vi "Configure Harmonics Fetch Step.vi"(6 "SA Pin":string="SA PIN", 8 "error in (no error)":errorcluster, 9 "Result Name":string, 10 "Harmonic Order":i8, 11 "Harmonics in":refnum<class "Harmonics.lvclass">) -> (0 "error out":errorcluster, 2 "Exported Data Location":string, 3 "Harmonics out":refnum<class "Harmonics.lvclass">)   [LabVIEW 2018, in "Harmonics.lvlib" / "Harmonics.lvclass"]
uses:
  Harmonics.lvclass
  C:/Sequence Automation/Plugins/Measurement Interface.lvlibp/Measurement Interface.lvclass
  Plugins/Measurement Interface.lvlibp/Private Methods/Engine Reference/Read Engine Reference.vi
  Plugins/Measurement Interface.lvlibp/Private Methods/Measurement Name/Read Measurement Name.vi
  Plugins/Measurement Interface.lvlibp/Public Methods/Sequence Reference/Read Sequence Reference.vi
  Plugins/TestStand API Tools (TSAT).lvlibp/Step Actions/TSAT Step Actions.lvlib
  Plugins/TestStand API Tools (TSAT).lvlibp/Sequence Actions/TSAT Sequence Actions.lvlib
  Plugins/Measurement Interface.lvlibp/Measurement Interface.lvclass
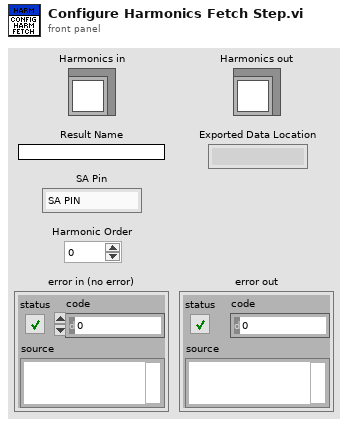
[diagram p1: front panel]
types:
  T1 = typedef "TestStand API Tools (TSAT).lvlibp/TSAT Evaluation Actions.lvlib/TSAT Evaluation.ctl" = cluster{"Test Name":string, "Pin":string, "Units":string, "SI Scaling":T2, "Test Number":i32, "Published Data Id":string, "Low Limit":dbl, "High Limit":dbl, "Export Data Location":string, "Software Bin":i64, "Evaluation Type":T3, "Test Data Source":string}
  T2 = typedef "TestStand API Tools (TSAT).lvlibp/TSAT Evaluation Actions.lvlib/TSAT Eval SI Unit Scaling.ctl" = i16
  T3 = typedef "TestStand API Tools (TSAT).lvlibp/TSAT Evaluation Actions.lvlib/TSAT Evaluation Type.ctl" = enum16{"Numeric Limit", "Pass/Fail", "None"}
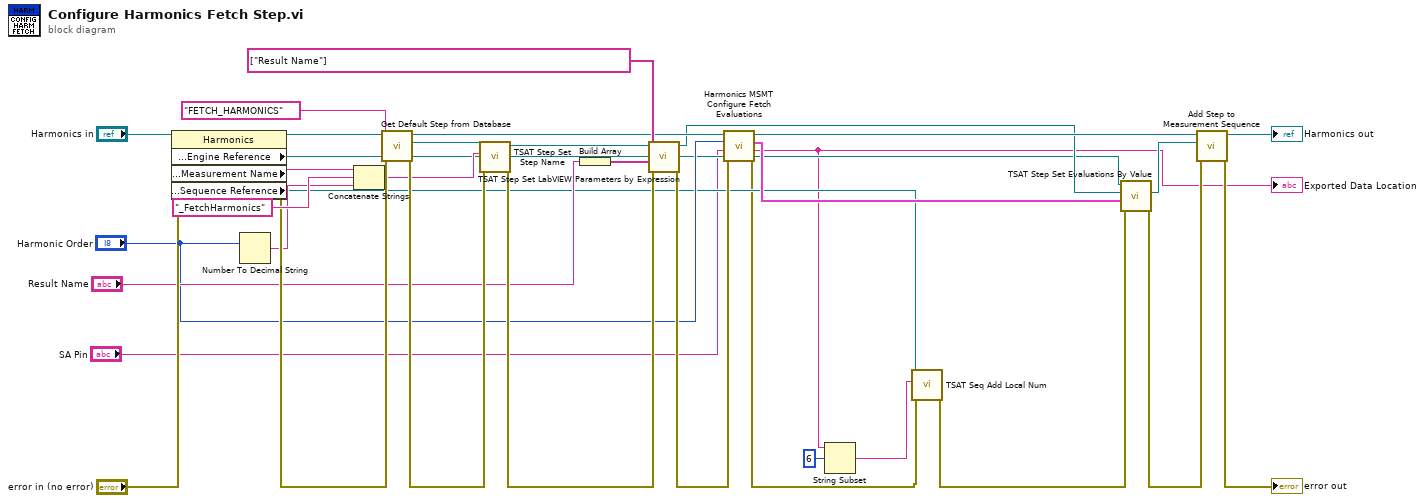
[diagram p0: block diagram]
diagram:
  n1 = property class="Harmonics"(reference="Harmonics in", error in="error in (no error)") -> (reference out=w27:refnum<class "Harmonics.lvclass">, error out=w28:errorcluster, "Protected Methods:Engine Reference"=w9:refnum<k7>, "Public Methods:Measurement Name"=w29:string, "Public Methods:Sequence Reference"=w7:refnum<k7>)
  n2 = Number To Decimal String(number="Harmonic Order") -> (decimal integer string=w25:string)  [unwired: 1 in]
  n3 = Concatenate Strings(w29, "_FetchHarmonics" ("string"), w25) -> (w18:string)
  n4 = call "Get Default Step from Database.vi"("error in (no error)"=w28, "Default Step"="FETCH_HARMONICS", "Measurement Interface in"=w27) -> ("error out"=w23:errorcluster, "Cloned Step"=w24:refnum<k7>, "Measurement Interface out"=w15:refnum<class "Harmonics.lvclass">)  [unwired: 6 in]
  n5 = call "TSAT Step Set Step Name.vi"("Error In"=w23, "Name"=w18, "Step In"=w24) -> ("Error Out"=w22:errorcluster, "Step Out"=w20:refnum<k7>)  [unwired: 7 in]
  n6 = Build Array("Result Name") -> (w16:string[])
  n7 = call "TSAT Step Set LabVIEW Parameters by Expression.vi"("Error In"=w22, "Value Expressions"=w16, "Parameters to Set"=string[] ["Result Name"], "Step In"=w20) -> ("Error Out"=w21:errorcluster, "Step Out"=w12:refnum<k7>)  [unwired: 6 in]
  n8 = call "Harmonics MSMT Configure Fetch Evaluations.vi"("error in (no error)"=w21, "SA Pin"="SA Pin", "Harmonic"="Harmonic Order", "Harmonics in"=w15) -> ("error out"=w6:errorcluster, "Exported Data Location"=w4:string, "Array"=w10:T1[], "Harmonics out"=w14:refnum<class "Harmonics.lvclass">)  [unwired: 4 in]
  "Exported Data Location" <- w4
  n9 = String Subset(string=w4, offset (0)=6) -> (substring=w2:string)  [unwired: 1 in]
  n10 = call "TSAT Seq Add Local Num.vi"("Error In"=w6, "Local Variable Name"=w2, "Sequence In"=w7) -> ("Error Out"=w5:errorcluster)  [unwired: 7 in, 1 out]
  n11 = call "TSAT Step Set Evaluations By Value.vi"("Error In"=w5, "Evaluation Data"=w10, "Step In"=w12, "Engine In"=w9) -> ("Error Out"=w8:errorcluster, "Step Out"=w11:refnum<k7>)  [unwired: 5 in, 1 out]
  n12 = call "Add Step to Measurement Sequence.vi"("error in (no error)"=w8, "Step to Add"=w11, "Measurement Interface in"=w14) -> ("error out"=→"error out":errorcluster, "Measurement Interface out"=→"Harmonics out":refnum<class "Harmonics.lvclass">)  [unwired: 7 in]
